vi "Save_Time_Traces.vi"() -> (5 "Plug in titles":string[](array[string]), 7 "Plug in values":string[](array[string]))   [LabVIEW 2016]
uses:
  Globals/Meas_global.vi
panel:
  in  "Channels to Save":T1(ring)=enum."All channels except Sync"
  in  "No of desired samples/ch":i32
  in  "Down Sample":i32=1
  in  "File Extension":string=".xls"
  in  "Full Header Info?":bool
  in  "Put each block into separate file":bool
  in  "Leave space between blocks?":bool
  in  "Precision":i16=2
  in  "Data to save":i32[](array[ring]) items=["FF (C)", "FF (C2)", "Save Nothing"]
  in  "Separation Character":enum16{"Tab", "Comma"}(ring)
  # "Run this VI to update the channel names"
  # "You Must have selected the \"Save Data\" option on the \nMeasurement Program for this vi to save time traces"
  # "0 means disabled"
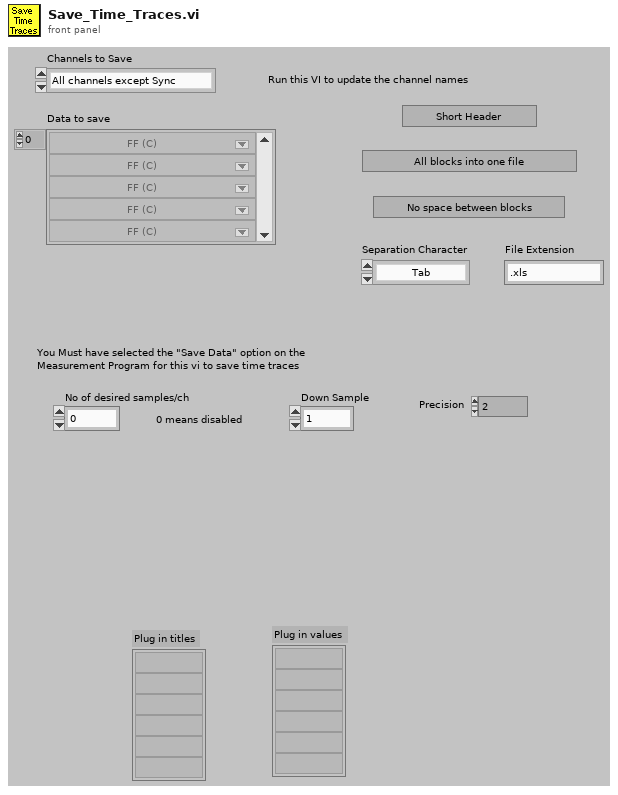
[diagram p1: front panel]
types:
  T1 = enum16{"Selected", "All channels except Sync", "All Channels"}
  T2 = typedef "Analysis_info_cluster.ctl" = cluster{"Colour":u32, "Inst type":T3, "Inst name":string, "Symbol":string, "Code name":string, "Extra Info":string, "Inst Array":T4, "Extra Titles":string[], "Extra Values":string[], "U":dbl, "u^2":dbl, "u^3":dbl, "u^4":dbl, "Skew_u":dbl, "Kurt_u":dbl, "Sd Error in Mean":dbl, "% u'/U":dbl, "X":dbl, "Y":dbl, "Z":dbl, "Timescale integral Estimate":dbl, "Sd Error in Variance":dbl, "Calib File":path, "Calib Constants":dbl[], "Output Position":bool, "Full Stats":bool, "Av Sampling Rate":dbl, "Av No of Samples":dbl, "Total Meas Time (s)":dbl, "ADAM Ch Name":string, "Max value":dbl, "Min value":dbl}
  T3 = typedef "Inst_type.ctl" = enum16{"Propeller anemometer", "Raw voltage", "Pressure Transducer", "Pitot-static tube", "Preston tube", "Hot wire", "Cross wire 1", "Cross wire 2", "Generic Linear", "Generic Polynomial", "Generic BackPoly", "Fast FID", "Thermocouple", "Cold wire", "Pulsed Wire", "LDA Vel", "LDA Tran time", "LDA Arr time", "Microphone"}
  T4 = typedef "Instrument_Array.ctl" = enum16{"PWA", "LDA", "Analogue"}
  T5 = enum16{"Save no data", "Save data in new files", "Save data in existing files"}
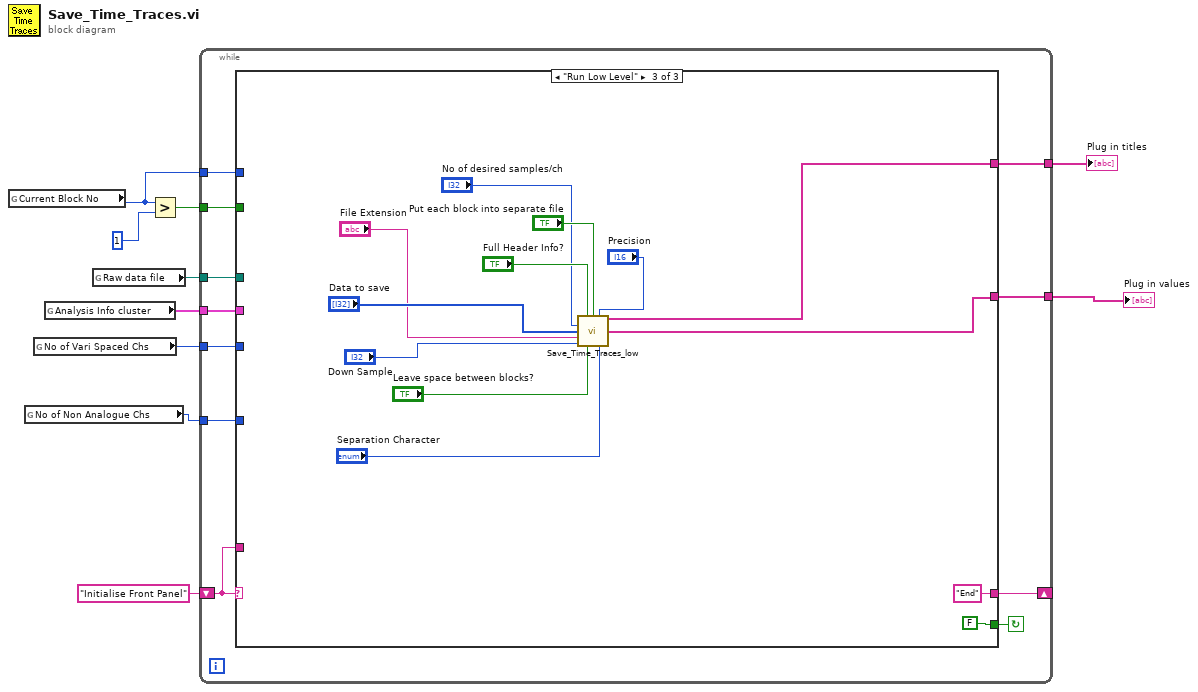
[diagram p0: block diagram]
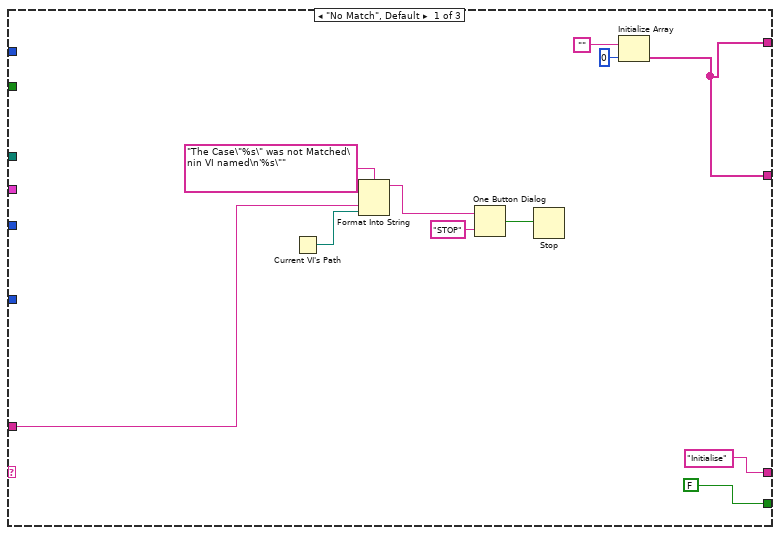
[diagram p2: hidden frame]
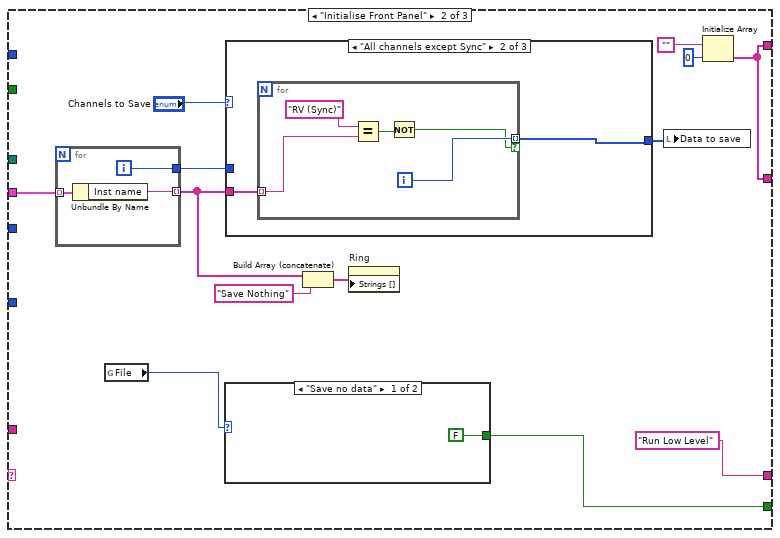
[diagram p3: hidden frame]
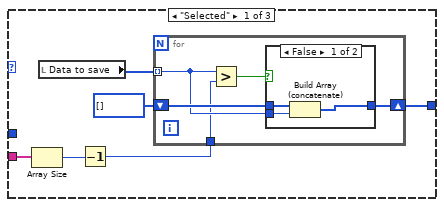
[diagram p4: hidden frame]
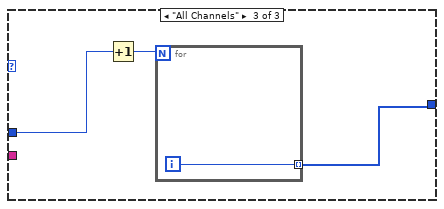
[diagram p6: hidden frame]
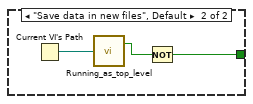
[diagram p7: hidden frame]
diagram:
  n1 = global read "Meas_global.vi" "Current Block No"() -> (w6:i32)
  n2 = global read "Meas_global.vi" "No of Non Analogue Chs"() -> (w3:i32)
  n3 = global read "Meas_global.vi" "No of Vari Spaced Chs"() -> (w4:i32)
  n4 = global read "Meas_global.vi" "Analysis Info cluster"() -> (w5:T2[])
  n5 = global read "Meas_global.vi" "Raw data file"() -> (w9:path)
  n6 = Greater?(x=w6, y=1) -> (0:w7:bool)
  n7 = while {
    shift-left: "Initialise Front Panel" -> [w19]
    shift-right: [w20] -> _
    tunnel: w9 -> [w18]
    tunnel: w7 -> [w17]
    tunnel: w6 -> [w16]
    tunnel: w5 -> [w15]
    tunnel: w4 -> [w14]
    tunnel: w3 -> [w13]
    tunnel: [w12] -> w2
    tunnel: [w11] -> w1
    stop <- w21 continue-if-true
    n8 = case shown="\"Run Low Level\"" w19 {
      tunnel: [FALSE w38 FALSE] -> w21
      tunnel: ["Initialise" "Run Low Level" ("t") "End" ("t")] -> w20
      tunnel: w19 -> [w27 _ _]
      tunnel: w18 -> [_ _ _]
      tunnel: w17 -> [_ _ _]
      tunnel: w16 -> [_ _ _]
      tunnel: w15 -> [_ w45 _]
      tunnel: w14 -> [_ _ _]
      tunnel: w13 -> [_ _ _]
      tunnel: [w22 w33 w79] -> w12
      tunnel: [w22 w33 w80] -> w11
      frame "No Match", Default {
        n9 = Current VI's Path() -> (path=w26:path)
        n10 = Format Into String(format string="The Case\"%s\" was not Matched\nin VI named\n'%s\"" ("Format String"), w27, w26) -> (resulting string=w30:string)  [unwired: 2 in, 1 out]
        n11 = One Button Dialog(message=w30, button name ("OK")="STOP") -> (true=w28:bool)
        n12 = Stop(stop? (T)=w28) -> ()
        n13 = Initialize Array("", 0) -> (w22:string[])
      }
      frame "Initialise Front Panel" {
        n14 = for {
          tunnel: w45 -> [w78] mode=indexing
          tunnel: [w77] -> w41 mode=indexing
          tunnel: [w76] -> w36
          i -> [w76]
          n15 = Unbundle By Name(w78) -> ("Inst name"=w77:string)
        }
        n16 = global read "Meas_global.vi" "File"() -> (w39:T5)
        n17 = case shown="\"Save no data\"" w39 {
          tunnel: [FALSE w73] -> w38
          frame "Save no data" {
          }
          frame "Save data in new files", Default {
            n18 = Current VI's Path() -> (path=w74:path)
            n19 = call "Running_as_top_level.vi"("Vi path name"=w74) -> ("Top Level"=w75:bool)  [unwired: 1 out]
            n20 = Not(x=w75) -> (.not. x?=w73:bool)
          }
        }
        n21 = case shown="\"All channels except Sync\"" "Channels to Save" {
          tunnel: [w49 w62 w69] -> w44
          tunnel: w41 -> [w46 w61 _]
          tunnel: w36 -> [_ _ w70]
          frame "Selected" {
            n22 = Array Size(array=w46) -> (size(s)=w48:i32)
            n23 = local read "Data to save"() -> (w51:i32[])
            n24 = Decrement(x=w48) -> (x-1=w47:i32)
            n25 = for {
              tunnel: w51 -> [w53] mode=indexing
              shift-right: [w54] -> w49
              shift-left: i32[] [] -> [w55]
              tunnel: w47 -> [w52]
              n26 = Greater?(x=w53, y=w52) -> (0:w56:bool)
              n27 = case shown="False" w56 {
                tunnel: w55 -> [w59 w60]
                tunnel: [w58 w60] -> w54
                tunnel: w53 -> [w57 _]
                frame False {
                  n28 = Build Array (concatenate)(w59, w57) -> (w58:i32[])
                }
                frame True {
                }
              }
            }
          }
          frame "All channels except Sync" {
            n29 = for {
              tunnel: [w67] -> w62 mode=indexing if=w63
              tunnel: w61 -> [w66] mode=indexing
              i -> [w67]
              n30 = Equal?(x="RV (Sync)", y=w66) -> (x = y?=w64:bool)
              n31 = Not(x=w64) -> (.not. x?=w63:bool)
            }
          }
          frame "All Channels" {
            n32 = Increment(x=w70) -> (x+1=w68:i32)
            n33 = for {
              N: w68 -> [_]
              tunnel: [w71] -> w69 mode=indexing
              i -> [w71]
            }
          }
        }
        n34 = Build Array (concatenate)(w41, "Save Nothing") -> (w42:string[])
        n35 = property on="Ring" class="Ring (strict)"("Strings []"=w42) -> ()  [unwired: 2 in, 2 out]
        n36 = local write "Data to save"(w44) -> ()
        n37 = Initialize Array("", 0) -> (w33:string[])
      }
      frame "Run Low Level" {
        n38 = call "Save_Time_Traces_low.vi"("Full Header Info?"="Full Header Info?", "Put each block into separate file"="Put each block into separate file", "Precision"="Precision", "No of desired samples/ch"="No of desired samples/ch", "Data to save"="Data to save", "File Extension"="File Extension", "Down Sample"="Down Sample", "Leave space between blocks?"="Leave space between blocks?", "Separation Character"="Separation Character") -> ("Plug in titles"=w80:string[], "Plug in values"=w79:string[])  [unwired: 2 in, 3 out]
      }
    }
  }
  "Plug in values" <- w2
  "Plug in titles" <- w1
